vi "Write Sequential Addresses.vi"(7 "Target IC (1-8)":u8, 8 "error in (no error)":errorcluster, 9 "Data":u16[](array[numeric]) format="%04x", 10 "Starting Address":u16 format="%04x", 11 "FPGA Sim in":refnum<class "FPGA Sim.lvclass">) -> (0 "error out":errorcluster)   [LabVIEW 2020, in "Unit Tests.lvlib" / "FPGA Sim.lvclass"]
uses:
  FPGA Sim.lvclass
  FPGA Sim.lvclass/FPGA Sim.ctl
  Dependencies/Virtual Memory Unit/Virtual Memory Unit.lvclass
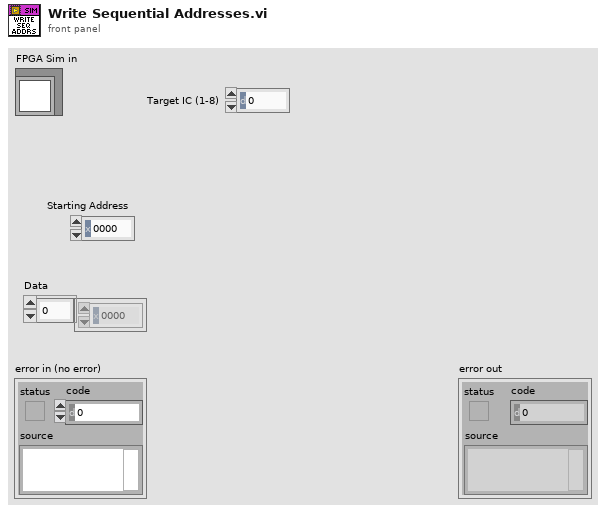
[diagram p1: front panel]
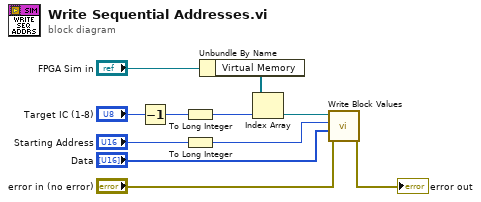
[diagram p0: block diagram]
diagram:
  n1 = Decrement(x="Target IC (1-8)") -> (x-1=w1:u8)
  n2 = To Long Integer(number=w1) -> (32bit integer=w10:i32)
  n3 = To Long Integer(number="Starting Address") -> (32bit integer=w5:i32)
  n4 = Unbundle By Name("FPGA Sim in") -> ("Virtual Memory"=w11:refnum<class "Virtual Memory Unit.lvclass">[])
  n5 = Index Array(array=w11, index=w10) -> (element=w7:refnum<class "Virtual Memory Unit.lvclass">)
  n6 = call "Write Block Values.vi"("error in (no error)"="error in (no error)", "Write Block"="Data", "Start Index"=w5, "Virtual Memory Unit in"=w7) -> ("error out"=→"error out":errorcluster)  [unwired: 6 in, 1 out]
